vi "Very Large Scan.vi"() -> ()   [LabVIEW 2020]
uses:
  Labview Library/Libraries/ASG8100CY/ASG8100CY.lvlib
  labview_control/LaoJi/NI CTR/NI DAQ Counter.lvlib
  Labview Library/Libraries/Actuator/Libraries/ActuatorXY/ActuatorXY.lvlib
  <vilib>/Utility/file.llb/Write Delimited Spreadsheet (DBL).vi
panel:
  out "Current Position Ref":refnum<vi>
  in  "Tab Control":enum32{"Main", "Page 2", "Debug"}(tab)
  out "Current Position":dbl[](array[numeric])=[99.99927521, 111.2070236, 118.3306351]
  out "Intensity Graph":dbl[][](graph)=[[12413.426204983658, 12199.09700975098, 13100.481023548917, 11916.694144612435, 12119.311516760476, 12635.21319012371, 12600.857673173667, 13200.126884929949, 12592.951932560312, 11969.74510595764, 12757.379319095471, 11664.809418891542, 11252.101294813838, 12673.211709104853, 12762.210663033009, 14052.009205428216, 12767.060980066512, 13491.678523119946, 12391.823407855252, 11682.597991673752, 13135.443159598599, 12561.438316974325, 12594.840161799231, 13137.006262002198, 12816.803806226804, 12264.51133348734, 13282.37239444406, 12068.37184342732, 13200.247759910138, 12739.193364141081, 12895.366092829376, 12574.704114298595, 13495.231009763791, 0.0, 0.0, 0.0, 0.0, 0.0, 0.0, 0.0, 0.0], [13918.401679718641, 13714.354354301113, 13034.107622027206, 12922.275529666118, 13284.51544235071, 13849.07101035678, 14229.907876224646, 12250.565796848681, 14368.52797214958, 11930.191715870234, 11958.175709508474, 13105.942468762929, 13127.623035352512, 13105.907908558916, 12944.940179229601, 12589.116808072462, 11930.893105657193, 12931.543845861952, 12948.5567459181, 13538.329558943446, 12206.628529994818, 12644.786069328475, 12145.374852409574, 13707.10706877193, 14002.386549620609, 13960.120590446573, 14233.993458009523, 12999.121140833002, 12498.726355937248, 13409.675547954475, 13890.523068108716, 13990.040985864322, 0.0, 0.0, 0.0, 0.0, 0.0, 0.0, 0.0, 0.0, 0.0], [12258.885994441494, 11540.699981915297, 12671.034725380556, 13626.04598248154, 12138.002922650432, 13724.579875024094, 13201.121594358172, 13406.793426249373, 12078.138573089063, 12625.023266417908, 11618.085489322053, 12985.45304949292, 13721.167006080777, 13294.601722768217, 12643.786506517528, 12910.677362525515, 12636.198302313776, 13450.034803844776, 13572.657979759677, 12959.536310430212, 14230.075367851714, 13101.468853699516, 13751.366005972177, 14847.158624393935, 14550.879575372923, 13469.328652192455, 12315.062611626825, 13303.949544773273, 12537.014442172915, 13137.644981314217, 12412.402936331515, 12742.456001832838, 0.0, 0.0, 0.0, 0.0, 0.0, 0.0, 0.0, 0.0, 0.0], [12694.372162417198, 13022.362890161545, 12661.942618493797, 13011.002050819809, 12568.862180133716, 12097.617475458834, 11886.783257923727, 13196.39299096777, 12574.726162508628, 13817.079693788166, 12952.933199438578, 11998.72639002685, 12725.850266025853, 12921.012420362225, 13116.183890060925, 12243.709381676368, 13406.677064262141, 12829.310502766873, 12819.63682004765, 14965.923746577075, 14282.102716657535, 14193.667647894785, 14001.343326690692, 14112.343845648364, 14258.49223877884, 13787.255521432566, 13900.845106555598, 13300.272018979244, 14621.216062749454, 13324.138114378447, 12753.532011624226, 13291.486009963373, 0.0, 0.0, 0.0, 0.0, 0.0, 0.0, 0.0, 0.0, 0.0], [12970.08256106479, 12755.433230499591, 12759.129541822067, 12131.866370843865, 13237.441493833365, 13004.551590371122, 12615.955472099551, 12489.827104668824, 13802.62250032107, 13201.604045018365, 13475.38636627498, 13263.586718391252, 12431.667821280345, 12146.212131205706, 11431.705474578237, 11935.857165786505, 13076.264149631565, 14053.653273820904, 13527.554378636914, 15083.728340807605, 14240.050392863022, 13712.466300859343, 13534.211849650283, 13916.161814929561, 13603.915208894614, 12724.175933694143, 14115.521428734177, 13699.377054098575, 12520.16952542519, 13143.571617498012, 12861.319494535608, 11964.754673245552, 0.0, 0.0, 0.0, 0.0, 0.0, 0.0, 0.0, 0.0, 0.0], [12837.099554190312, 13730.039481956715, 13729.236149582926, 12773.22315006938, 12449.36205497966, 12785.572491273708, 12764.465845887613, 12994.325806181272, 12714.702145013536, 13238.071134532476, 12915.19688512138, 13249.255351726322, 14121.254504473844, 12260.006974490901, 12593.537750831047, 13058.366060936138, 12230.519744388814, 13649.845877797894, 14208.99419364147, 13172.418622381581, 14028.88379983732, 14304.007844736365, 12729.821623627164, 14018.217130770625, 12876.63311433904, 13339.02464907911, 13686.55164368562, 12653.270268864537, 11687.751773397524, 14504.962939666611, 13514.353683396563, 12698.999482473548, 0.0, 0.0, 0.0, 0.0, 0.0, 0.0, 0.0, 0.0, 0.0], [13835.660926920731, 11722.788966750355, 13769.097382965234, 13678.968748706233, 13089.742611497875, 13408.31701152738, 12433.082271814066, 13644.416984836844, 12930.603615104978, 13441.534344950353, 12074.964570721304, 13998.007066951823, 13140.736615945742, 11457.928449629886, 13243.337051247401, 13132.571799008621, 13556.25847025227, 13266.56825136083, 13759.25276363223, 13222.940798425003, 12226.586254185257, 12399.172944289516, 12940.666377460031, 12378.023558911598, 12735.176254639584, 13256.409423687672, 12502.46312201368, 12641.192647307607, 13864.041481336862, 10910.96844711718, 12951.07038744892, 13897.890596552874, 0.0, 0.0, 0.0, 0.0, 0.0, 0.0, 0.0, 0.0, 0.0], [13267.677925089234, 14283.60175716499, 12335.566256102135, 13295.740020797984, 13540.983823787685, 13071.811249785284, 13279.048757437493, 12658.988883489092, 14360.12103870256, 12765.068844317735, 12462.974160932763, 13449.15481857287, 12483.51941953124, 13571.643726880155, 12881.600996229157, 11701.869219834029, 13048.415806461859, 12637.200253227616, 13986.802023347125, 12709.817363228733, 13055.41945281852, 12432.331894928056, 12696.068428366405, 12886.427182168558, 12978.607208713736, 12200.297054732728, 13006.564731219401, 12985.287768575094, 13518.967571938578, 12506.537507612435, 11267.832353948912, 11994.032241170093, 0.0, 0.0, 0.0, 0.0, 0.0, 0.0, 0.0, 0.0, 0.0], [13947.00139457789, 13331.572961523247, 12915.551134096198, 12670.150399341737, 13018.4849369988, 13851.488791463342, 12911.337638456574, 12843.950999847997, 13558.792150795012, 12799.452431282652, 12923.843316135377, 13011.771113391505, 12634.113427980472, 14059.777594765874, 12752.741503344181, 13751.440184666115, 11876.017007412478, 12536.136490651717, 12907.728373486574, 11110.785279296422, 12224.148192732144, 12881.137035175328, 11652.240083657447, 12261.757631216198, 12654.62158363913, 12837.346905705253, 13604.085733591222, 12992.350424055434, 12590.268312446482, 13552.180822354245, 13018.53918713744, 13181.501959240637, 0.0, 0.0, 0.0, 0.0, 0.0, 0.0, 0.0, 0.0, 0.0], [12537.114237940512, 12761.908436904923, 12729.829897669371, 13253.403017391156, 13096.430570004553, 14105.53717241387, 11077.027950579277, 12762.431676759352, 13806.015378703643, 12836.928438252402, 12884.267634496216, 12355.610774069048, 12534.66407270051, 13849.386237015919, 14946.701049975214, 12845.299773218543, 11793.55286062109, 13653.118236811586, 12506.03796888722, 12454.347540059242, 11370.323456376876, 12289.249415225073, 11926.627389740292, 12878.692883758606, 13467.001048772585, 13034.782634630774, 13442.312889726498, 13518.001076147912, 14420.255986287922, 12821.079626999623, 12707.021281232992, 12766.684649955621, 0.0, 0.0, 0.0, 0.0, 0.0, 0.0, 0.0, 0.0, 0.0], [12487.381516153826, 14339.319214684385, 12952.083892837984, 13042.298089558928, 11814.040971125112, 12993.245469552056, 11824.266928359524, 12704.546508075906, 12378.064320131107, 13955.37634137259, 13222.720190755503, 12842.786688775011, 12781.837874872224, 14230.39468332686, 13776.254622417897, 12565.57764822756, 12802.501202154437, 13481.234256200964, 13121.367591580052, 12214.942948555188, 12572.122074449308, 12294.665541499931, 11647.169328782516, 13389.589848651389, 13145.55231421336, 13022.516033877246, 12531.205641182538, 12454.90174430176, 13651.922591104285, 13244.0219322327, 13714.922110203477, 13115.428630787026, 0.0, 0.0, 0.0, 0.0, 0.0, 0.0, 0.0, 0.0, 0.0], [13871.946798881001, 13137.465659369618, 12438.056502485917, 12421.185781436325, 12632.60075176157, 12675.161365119719, 12398.995128619465, 13758.94331665558, 12771.263310990475, 12660.486821039187, 12813.183122209603, 12039.442258650037, 13034.033306046578, 13007.094176496232, 12806.719300435076, 13292.78429470634, 11376.872444320257, 13765.106623258476, 12035.178724409687, 13982.013021054343, 13945.65520895236, 12099.577516209834, 12636.400730915822, 12800.802138670857, 13540.83288539829, 12760.59903885621, 12539.225480698393, 14033.338568510966, 12267.604342318273, 12832.589310804566, 12829.312409175322, 12135.672708799944, 0.0, 0.0, 0.0, 0.0, 0.0, 0.0, 0.0, 0.0, 0.0], [12455.858749892846, 12623.133379160781, 12500.86582954595, 12528.366879721654, 11695.349738708808, 13057.094185604197, 12918.713824075225, 13429.752062168367, 13144.681572748195, 14062.331790855842, 14133.900456575315, 13562.371687492217, 13879.543762425294, 13539.298808378722, 12813.118537834911, 11878.981212560637, 12238.440644268509, 13285.492309722144, 12456.477873719256, 11602.41926149364, 14161.420151438455, 13038.032144165492, 12766.45508319012, 12633.416033100453, 11593.70075901844, 12961.846388662292, 11534.410992302064, 12680.87149702491, 12570.498986741186, 12400.744702794887, 12473.300881067033, 11578.738839559071, 0.0, 0.0, 0.0, 0.0, 0.0, 0.0, 0.0, 0.0, 0.0], [13273.618931821715, 13609.664480714086, 12495.912926045647, 11807.334082303123, 13623.978204541841, 12496.801019503186, 13423.36755685845, 13658.982940375161, 13151.711243542646, 13707.132022575093, 15030.21072087198, 14811.975611139635, 13935.041268841054, 13344.116461784426, 13974.194321770477, 13058.07100568908, 11872.978591312276, 12633.960630367956, 13874.030490294443, 13223.140501311796, 13449.693043326033, 12865.093964362582, 14573.210778783121, 12937.89151870477, 13528.587269419117, 12326.29996655928, 13291.441050661637, 12537.612837597128, 12336.303662429049, 13178.792282272538, 12854.311264287297, 11531.867412501098, 0.0, 0.0, 0.0, 0.0, 0.0, 0.0, 0.0, 0.0, 0.0], [13559.475618266475, 12708.238154432383, 13325.441673780018, 12580.807494439696, 12774.39398446758, 13169.667542076919, 12512.951566178062, 13328.069590584042, 14049.434961167764, 14034.014646536674, 14249.950611104257, 13662.509612307922, 13536.090560109578, 13444.830360467091, 12999.22646787052, 14296.542926343876, 13778.174702169568, 13598.705918248295, 12922.431587196003, 12819.663440612918, 14154.671366562798, 11879.250121768884, 12489.774206606979, 13007.187654857686, 12682.65963905539, 13374.869918322547, 13000.101772810256, 11466.189567113694, 11687.54615721876, 13263.679227321192, 12554.14606653799, 12744.765064601508, 0.0, 0.0, 0.0, 0.0, 0.0, 0.0, 0.0, 0.0, 0.0], [12057.281754790905, 13387.018005800162, 12870.58405669512, 11434.570515641148, 13046.61228460777, 12890.555140926346, 14074.4996600198, 13598.584666875637, 13943.588802829441, 14577.02596700239, 14899.311664954468, 14125.407337372551, 13767.921744085745, 14284.758467923384, 15150.342978651532, 13758.234606286367, 15287.521726844541, 14210.937685664203, 13071.850929958635, 13162.13602627519, 13156.529223939751, 13754.827910812202, 14063.703872320904, 12580.05864518567, 12815.970416069284, 13279.850720117265, 14251.8788873906, 15911.396908698733, 12792.9727551923, 14541.243511556966, 12623.955055396002, 12233.341117493372, 0.0, 0.0, 0.0, 0.0, 0.0, 0.0, 0.0, 0.0, 0.0], [12422.400854292599, 13006.101586817997, 12270.677099054536, 12788.713622996089, 13069.934150232626, 13427.738445826217, 13197.712398815935, 14806.48232783516, 14093.664993931981, 15246.832539050914, 13706.140353533836, 15044.001245140858, 14574.332330867643, 15451.759803052615, 14425.683852177626, 14999.999995469241, 14492.149549680014, 14794.979291817484, 14502.670743306082, 13371.240573606086, 13123.269879924728, 13982.645466003423, 11868.955939150304, 13309.303570999804, 12085.546335378644, 13774.74630045686, 12561.019938546375, 14103.989803286822, 12943.419711271907, 14838.47766353947, 12259.99290706767, 13533.39019912427, 0.0, 0.0, 0.0, 0.0, 0.0, 0.0, 0.0, 0.0, 0.0], [12865.076239061886, 12983.967180450174, 13122.511901548021, 13270.715956288306, 13316.070515659632, 14889.493068517446, 14754.714918544232, 15703.222518057488, 15584.692963321164, 15170.03076251474, 15265.426330695644, 14620.072198552392, 14710.705696304709, 14920.583460947415, 15090.151819254193, 15905.83202339489, 14811.806842630936, 14907.515195633481, 13706.047582468886, 14097.047042284901, 13755.202393529396, 14914.267983744412, 13509.689238613517, 13215.87365729284, 14479.769644192691, 13650.401067511768, 14133.66599702661, 14185.046211909372, 13395.981871932736, 13209.642036389812, 13184.931504820266, 11385.65343361341, 0.0, 0.0, 0.0, 0.0, 0.0, 0.0, 0.0, 0.0, 0.0], [12557.855834145807, 12405.97320016197, 13248.758142845036, 12191.34347029364, 14140.106775683014, 14758.926276562219, 15453.21646644145, 15676.658868274886, 14223.4472983029, 16420.85750820729, 14955.950307825911, 15901.80130348282, 15280.378695010344, 15898.304741990773, 15643.332032499364, 16967.81166005398, 15653.588130649729, 14133.05868971342, 13631.134842905734, 15411.594102522207, 14742.377789088294, 14610.103269986652, 13456.5785056317, 13242.281827083545, 14994.206024423704, 14225.606086375425, 14706.421803722222, 15220.649014973435, 12800.431173191871, 13296.491672940598, 13480.498208474472, 12429.374756756852, 0.0, 0.0, 0.0, 0.0, 0.0, 0.0, 0.0, 0.0, 0.0], [12502.114084437491, 12088.404760758222, 13006.384657046532, 13164.00292053339, 13958.505173627442, 14051.552437733617, 13182.061549729364, 15677.026458255068, 15357.841051746631, 14787.809816088495, 16070.697535450803, 16623.275823499192, 14695.645447177383, 16777.92568969485, 14748.60477751724, 15776.157172708974, 15966.767470527393, 14344.047394303958, 15180.2530425606, 14022.757696580164, 14318.918281398463, 14449.611400859467, 13568.738138656865, 14758.521208606704, 13373.508088178725, 13261.572740959322, 14190.787256041518, 13844.008296598327, 13911.94936060347, 12588.100731247758, 14264.334488316377, 12266.928359111278, 0.0, 0.0, 0.0, 0.0, 0.0, 0.0, 0.0, 0.0, 0.0], [12643.366747476926, 11972.530949574875, 13215.254758431174, 14143.841857093452, 12998.965454429928, 13086.238313848029, 15228.324013017324, 15066.738129939753, 16109.733354191218, 15386.56662902939, 16654.96137158211, 17019.565805166, 17304.700496789676, 17078.416436532407, 15632.53884190061, 16197.871133421206, 16829.430171183158, 15584.499221002216, 16292.25163612787, 15966.85228224687, 15275.794506995153, 14030.78736369024, 13084.90193058179, 13254.393049800092, 13753.271002236645, 14077.399983315414, 12308.73432053298, 12926.175679519885, 14349.056090635228, 13604.18653151363, 14535.72137306923, 14496.984491907573, 0.0, 0.0, 0.0, 0.0, 0.0, 0.0, 0.0, 0.0, 0.0], [13370.31128965041, 12977.621033955824, 13245.828564228366, 13493.345323087793, 12392.031485138597, 14437.06914668699, 13851.933787126258, 13990.125805728161, 15128.28720743473, 16031.996202895887, 18481.02026150857, 15242.041644692315, 15475.064201506602, 17548.89108099867, 16827.477646509346, 16001.075702118389, 16024.746412389559, 13721.732727761864, 15622.605805381503, 14467.708881398506, 13811.451629723742, 13880.69199344368, 12927.203687720485, 13349.719588084066, 14861.525356985228, 13272.498346911241, 13202.3354016208, 13737.22916825854, 14822.79564942803, 12780.848688908936, 14063.755691859693, 12791.479310696497, 0.0, 0.0, 0.0, 0.0, 0.0, 0.0, 0.0, 0.0, 0.0], [13517.048924991845, 13100.303643349873, 13839.567226684294, 12142.645485765588, 14453.177249270428, 13688.116915307666, 15547.253147175443, 15954.827490843272, 15715.610837607983, 16690.100248954266, 16737.182882883866, 17332.371926015054, 17483.445469268157, 18032.64214448167, 16258.530707332775, 18352.657472328567, 17106.21525641404, 15463.91752196599, 14996.20028311758, 14695.650700387292, 14185.583457328059, 14440.905008296115, 14744.970853913053, 14118.372997513872, 14936.7181012185, 13771.121924452144, 14314.451070459847, 12855.118432209549, 14354.051659138218, 11967.120500064968, 14193.924072474974, 13247.640785598678, 0.0, 0.0, 0.0, 0.0, 0.0, 0.0, 0.0, 0.0, 0.0], [12293.471357192411, 12226.38799955064, 12455.913516216571, 13132.266009733257, 12515.153790258608, 14031.228647166721, 13407.083294154087, 15968.0, 14507.309454949069, 14583.57069331596, 17753.48118832408, 16535.883876102675, 16794.35978579401, 17636.564434961343, 16603.89990629336, 17441.3154992632, 16269.796786663635, 16473.734108182693, 15696.2257062951, 16975.724388869025, 15210.370341047173, 14811.325017684518, 13664.979709970776, 13856.540583741911, 13489.57623695918, 12631.305501319124, 13405.634386460397, 13359.416003160526, 13953.347283944195, 12697.303672809827, 12462.095868575663, 12778.664271419344, 0.0, 0.0, 0.0, 0.0, 0.0, 0.0, 0.0, 0.0, 0.0], [12739.955228234921, 12252.907673381264, 12801.7679899394, 13294.090413170095, 14134.60390237021, 13991.282354129253, 14271.27311981502, 15407.413222724821, 15513.094778385946, 15822.784812125014, 15958.382134633239, 17960.3805298721, 17428.25201286278, 18646.49192184965, 18010.136260562962, 17987.698732719633, 16621.851214287206, 17419.350675631824, 14746.729957890026, 16777.484940513015, 14663.050448157548, 15149.769193942475, 13594.50468167116, 12971.95571029519, 13366.16250299396, 12349.151681346619, 12725.143669905005, 12272.261648545456, 13121.273709971618, 12879.967441739718, 14028.928847064983, 13068.977678399828, 0.0, 0.0, 0.0, 0.0, 0.0, 0.0, 0.0, 0.0, 0.0], [12492.171790246337, 12551.296234250594, 12523.838945963844, 13092.18518370972, 13189.210632081813, 13993.311673674876, 15138.365318643078, 15881.48765545004, 14969.463622618972, 16971.054736996215, 17380.43377702291, 17703.209709159855, 18240.090037959006, 18556.175213247105, 19058.00821273062, 17323.793468892956, 17680.666059191233, 17778.0737066739, 16422.91368294277, 17404.177001192867, 15637.16410537616, 15125.235586627014, 13553.18135902796, 13446.839145489132, 12768.609994172646, 13309.477355584726, 12447.648129482914, 13631.593915719834, 13284.350702105781, 12139.353126605076, 13480.154400361962, 12872.839321693937, 0.0, 0.0, 0.0, 0.0, 0.0, 0.0, 0.0, 0.0, 0.0], [12501.218197771126, 13324.561608671956, 13544.228395442931, 14816.710555904923, 13244.515887114781, 13765.09746853085, 13594.702454196735, 14350.176707978415, 16495.896145625025, 15799.358089614818, 17181.378087997113, 17537.402994756165, 17962.282492253744, 18119.663872488527, 18263.633347809395, 18213.93801668653, 17843.268935628905, 18433.51645479146, 17704.723103492543, 16231.087584686296, 15342.895878798776, 13927.251761496851, 14212.715865666474, 13157.983069318136, 12595.594549627556, 12725.481646331766, 13662.128444131216, 11230.395636643447, 12706.649815223052, 11858.055682181477, 12769.603673594662, 13256.05472940554, 0.0, 0.0, 0.0, 0.0, 0.0, 0.0, 0.0, 0.0, 0.0], [13857.512544698839, 15709.216972577115, 13848.000592018663, 14110.679397444079, 14756.817814177983, 15096.268528199036, 12735.728593020624, 15320.003168173227, 15090.273969405855, 16005.173919122013, 17046.84089677335, 17393.15289041886, 18125.610479449595, 17787.264316011195, 18970.794026374908, 17624.76965585236, 18281.067410376992, 17661.230722608478, 17205.415389510803, 17345.302984928276, 15212.671105467827, 14688.767236535048, 13946.495567374315, 12844.060685767745, 14040.530987236269, 12518.146398162238, 13168.142994125754, 11890.997005219937, 13168.236986434023, 12623.06657443203, 13513.603693615176, 12036.432468689562, 0.0, 0.0, 0.0, 0.0, 0.0, 0.0, 0.0, 0.0, 0.0], [13097.880192123343, 14864.981970879613, 14627.456956976983, 15552.256928214605, 13415.88917238188, 14236.363461612693, 15100.844916793774, 14324.58574553272, 14207.116537719327, 15266.91659575524, 15376.036476378296, 15405.55198621008, 19277.719226439214, 19088.18477521673, 18259.14035344528, 16354.43568518216, 18061.994943115293, 16189.680383339952, 15352.895826718584, 16828.268842122066, 16167.988698654633, 13773.789233408259, 14189.928754118526, 14367.526706090597, 13246.187950383897, 12517.900594985009, 13030.919715266717, 12732.443078431555, 12235.79495883463, 12999.07149635248, 12005.301542396843, 14455.123105077117, 0.0, 0.0, 0.0, 0.0, 0.0, 0.0, 0.0, 0.0, 0.0], [15246.179965103964, 14126.293675762003, 14031.191647729174, 14275.37329256934, 14816.681877770283, 14557.588893472044, 15688.30788989457, 15037.544288471167, 14222.45101272904, 16366.998724887004, 16421.526389762777, 16420.862637726277, 17119.8488130454, 16819.05262691617, 16177.10235398821, 16385.846391456893, 17035.060610621113, 15480.290211366118, 16175.113479403877, 15480.599207516281, 15536.325493579932, 13836.713632696987, 14908.564031588003, 13717.196582080323, 14121.089185366753, 13685.977604640037, 12703.507919690355, 11598.961746518808, 12696.99762924022, 13991.394101252918, 13340.020054818053, 13616.001980236257, 0.0, 0.0, 0.0, 0.0, 0.0, 0.0, 0.0, 0.0, 0.0], [13348.497950252045, 13506.750167273307, 15028.604443487327, 14246.884724386808, 14043.850657356252, 13900.207677924574, 15267.328915390899, 15791.751767201928, 13885.804993337651, 13930.163446078157, 15603.73273743012, 15300.516986772584, 15471.739280942544, 16342.76219366645, 17728.242759781242, 15403.447926612622, 15525.039055321551, 13232.790721734305, 16693.36707555501, 16196.668202975228, 14115.605511000507, 14334.102073947297, 13834.184535360573, 13883.961471756236, 13733.511707205587, 13118.601385081918, 12431.922343075488, 12413.14001388472, 12252.29604100895, 12440.270750048076, 13576.253284341266, 11599.913926930345, 0.0, 0.0, 0.0, 0.0, 0.0, 0.0, 0.0, 0.0, 0.0], [13729.208643133363, 13505.537267109772, 14952.454555642722, 12824.219742429017, 13948.172205462286, 14768.646225242834, 15143.051353850638, 14688.501299425247, 14210.60110649001, 13442.568131046195, 13605.711100217126, 15635.372330016322, 15971.686857426057, 15354.789714392211, 15062.971126506165, 14566.813116735319, 13300.194803027896, 16243.168211692695, 15535.322671806609, 13612.768577859002, 14605.23411064778, 13027.183819050211, 13723.649400282351, 13395.438482473251, 13091.934101877308, 13302.805954408203, 14096.904415798377, 13461.631139376794, 11324.32201534619, 12200.838651300497, 12664.751235145191, 11712.942296521996, 0.0, 0.0, 0.0, 0.0, 0.0, 0.0, 0.0, 0.0, 0.0], [15029.384806434518, 12569.01736952105, 12846.287523674122, 13173.628422471333, 12887.905670652466, 14366.09601363714, 15233.979154066246, 14600.939878666115, 15520.215253866694, 14334.097817974744, 14761.325334436333, 13450.035484390155, 15354.646500560337, 14764.68778317609, 14904.555301160555, 14029.040110133781, 16387.544164082676, 14799.202471458559, 15024.018662889535, 14995.83075037572, 13420.125581345952, 14816.24848076997, 12784.69624422291, 14188.507311587497, 12794.962400314433, 13284.66673254992, 13554.669363184932, 12495.763419630362, 13922.799084791932, 11726.766342883966, 12733.805008298104, 13625.490774379878, 0.0, 0.0, 0.0, 0.0, 0.0, 0.0, 0.0, 0.0, 0.0], [13727.31503077312, 12282.896552873406, 12993.606742294905, 13184.689656000468, 12685.114166978861, 12564.88216091661, 14120.030322701125, 13648.51032068617, 15312.047857923608, 15928.75268809039, 13705.80473244243, 14340.57159037476, 15814.613995717678, 15144.30647461296, 15688.840229551712, 13648.967072039415, 12962.013565685227, 14799.86318057995, 15426.082509773065, 13895.609640377876, 12950.463641557633, 14589.661495547989, 14854.446588357481, 14610.151893552327, 13295.207049484869, 13549.85940445823, 12465.947921569084, 13438.51208756311, 13113.695743245058, 11811.299477059334, 12788.055827456903, 12920.631843040062, 0.0, 0.0, 0.0, 0.0, 0.0, 0.0, 0.0, 0.0, 0.0], [12804.946825551533, 12791.199653148495, 12071.699812420959, 13917.748703517744, 14236.049170355049, 12523.140583219623, 14135.593218330794, 14016.926350128426, 14782.670899585271, 13977.399254413027, 14945.141189508104, 16076.411828437103, 14750.01444149086, 14732.196699167493, 14139.271832119426, 14085.960995176261, 14305.177111496541, 14257.64952428444, 14344.058172141422, 14803.254030985618, 12904.036974235898, 13383.77647676246, 14250.589598657838, 13180.8856912157, 13834.270131972404, 12623.944177430141, 12899.683461629096, 11931.100401709418, 11859.329608688635, 12815.519762479062, 12735.252931866487, 11843.702928989931, 0.0, 0.0, 0.0, 0.0, 0.0, 0.0, 0.0, 0.0, 0.0], [12957.404586111807, 13666.056251335754, 12980.101503702803, 13188.998346504977, 13127.206869172911, 14144.745660879502, 14050.312859386764, 15716.274822710113, 16041.235603585264, 14735.315637686552, 14984.983065197728, 15420.7910922481, 14813.1073984849, 15540.56799316592, 13642.796874114263, 14362.742429601447, 14840.663418430944, 14491.688977238939, 14224.175705007425, 14071.3259096335, 13661.24837889464, 15026.090761876205, 15260.121626611746, 13753.46334192511, 13705.96708397043, 12838.055241430058, 13377.426777450231, 12404.63106190544, 12733.703890280683, 13024.602027687073, 12480.015108382144, 11631.777053228614, 0.0, 0.0, 0.0, 0.0, 0.0, 0.0, 0.0, 0.0, 0.0], [13002.804843208633, 11811.565261822558, 13489.585009489738, 13811.572545480136, 13302.54419753063, 14220.282092638818, 14689.239132242525, 13064.070167676142, 13965.107572837285, 14460.1323299737, 14568.164861466355, 14574.662758239338, 13479.822798288506, 13532.303298792694, 13056.10095574842, 14442.509120502398, 15247.03913809049, 15083.723142365574, 15233.089918630953, 13259.410173035287, 13127.524042032166, 14663.782789333141, 14458.587662937818, 13538.805881771654, 13571.853268003166, 13217.732697251353, 13544.077857824113, 14047.523485774134, 12554.59064996008, 12026.359142968025, 12307.24916444649, 12116.711290398584, 0.0, 0.0, 0.0, 0.0, 0.0, 0.0, 0.0, 0.0, 0.0], [13222.635289906524, 11091.529371599912, 13004.251650159811, 12852.337155803456, 14024.911234078503, 13591.217981810014, 13793.944896941335, 12951.210306527455, 12949.281982647923, 14055.745620423138, 14044.395893315319, 15416.551159652292, 13513.118446796138, 13280.30066852846, 13652.56574197326, 14650.778114125224, 14976.165381280407, 15812.766128024667, 14269.985464336123, 13641.291932379732, 14942.374695675784, 14058.667517009784, 14206.669659525169, 13652.907534170503, 15058.624562195728, 13640.069067117907, 13035.234632089787, 10818.666763440126, 11304.677389605513, 11759.716226476483, 12100.433601076704, 11103.246776798322, 0.0, 0.0, 0.0, 0.0, 0.0, 0.0, 0.0, 0.0, 0.0], [12645.894926423447, 12482.962444657896, 12076.153979506542, 12662.77656720931, 12794.792006336971, 12355.777956527543, 14132.759393395849, 13598.726756561999, 13736.358552396936, 13877.493136245925, 14506.251967335653, 14208.245512601516, 13972.98556176245, 13635.745381158742, 14767.05691273909, 14805.378724277194, 15834.015833377387, 13517.302141320668, 15438.58245449284, 13395.824913848006, 14824.064394724826, 14845.036338921109, 13350.223134307002, 12718.91204373206, 13342.668799214853, 12785.967484737008, 11633.879760877078, 12180.776869167603, 13092.33853423821, 11411.078997047905, 11698.363197843963, 10903.754834233272, 0.0, 0.0, 0.0, 0.0, 0.0, 0.0, 0.0, 0.0, 0.0], [12762.876532702567, 13762.795366723818, 11916.017978444854, 12386.960953703696, 13156.515184616015, 13124.633795523241, 12944.67675822541, 10643.513263982872, 13206.96084170968, 12076.80714930371, 13954.7771756304, 13330.282621758099, 13880.01277806489, 14093.834373576548, 13585.69592239855, 13462.574042706883, 14746.456093046532, 15411.092592219895, 14793.35426580775, 14648.48649056882, 13936.955379988762, 13237.331327400436, 14454.292055706217, 14312.830772530475, 13258.381066170188, 11968.373655259922, 11928.455200175982, 12776.501995674073, 12735.262754400004, 11778.916736678044, 11382.856259846201, 12790.643025596868, 0.0, 0.0, 0.0, 0.0, 0.0, 0.0, 0.0, 0.0, 0.0], [13135.83545562699, 13463.141813472537, 13303.099015686603, 12086.433056971766, 12390.042434642626, 13095.792063255712, 12981.998291371598, 11827.72134134359, 13314.808382104955, 13008.566207053842, 13867.574526491906, 14878.16079937208, 14060.921713992824, 14044.237671271945, 13406.866004176907, 12793.490351395216, 14926.971628422307, 14568.431249999461, 15010.428470300994, 13720.299050346766, 13390.56362915429, 13164.628559875404, 13031.943261949038, 14671.44895724443, 12978.231819887067, 12770.45031559331, 12044.766378340522, 12134.138631367123, 12158.41820615577, 11684.524463787544, 11831.95958540421, 12009.08249742605, 0.0, 0.0, 0.0, 0.0, 0.0, 0.0, 0.0, 0.0, 0.0]]
  in  "Scan parameter":T1={"Horizontal axis"=0, "Vertical axis"=1, {"horizontal start"=100.0, "horizontal end"=104.0, "horizontal num"=40, "vertical start"=108.0, "vertical end"=112.0, "vertical num"=40}}
  in  "Stop Button":bool
  out "count Rate":dbl=13495.231009763791 format="%#.1f"
  in  "Pause Button":bool
  out "Laser On":bool
  out "Read + Move Time":u32=53
  in  "Sample Rate":dbl=25.0
  in  "Store path":path=path "I:/scan map test"
  out "vertical range":dbl=4.0
  out "horizontal range":dbl=4.0
  out "horizontal step":dbl=0.1
  out "vertical step":dbl=0.1
  out "Horizontal axis":i8(ring) items=["x", "y", "z", ""]
  out "horizontal end":dbl=104.0
  out "vertical end":dbl=112.0
  out "horizontal start":dbl=100.0
  out "vertical start":dbl=108.0
  out "vertical num":u32=40
  out "horizontal num":u32=40
  out "Remain axis":i8(ring)=2 items=["x", "y", "z", ""]
  out "Vertical axis":i8(ring)=1 items=["x", "y", "z", ""]
  in  "Stop Signal Ref":refnum<vi>
  in  "Scanning":refnum<vi>
  in  "Intensity Graph Ref":refnum<vi>
  out "Position After move 2":dbl[](array[numeric]) format="%.6f"
  out "Position After move":dbl[](array[numeric]) format="%.6f"
  out "V goal position":dbl[](array[numeric])=[108.0, 108.1, 108.2, 108.3, 108.4, 108.5, 108.6, 108.7, 108.8, 108.9, 109.0, 109.1, 109.2, 109.3, 109.4, 109.5, 109.6, 109.7, 109.8, 109.9, 110.0, 110.1, 110.2, 110.3, 110.4, 110.5, 110.6, 110.7, 110.8, 110.9, 111.0, 111.1, 111.2, 111.3, 111.4, 111.5, 111.6, 111.7, 111.8, 111.9, 112.0]
  out "H goal position":dbl[](array[numeric])=[100.0, 100.1, 100.2, 100.3, 100.4, 100.5, 100.6, 100.7, 100.8, 100.9, 101.0, 101.1, 101.2, 101.3, 101.4, 101.5, 101.6, 101.7, 101.8, 101.9, 102.0, 102.1, 102.2, 102.3, 102.4, 102.5, 102.6, 102.7, 102.8, 102.9, 103.0, 103.1, 103.2, 103.3, 103.4, 103.5, 103.6, 103.7, 103.8, 103.9, 104.0]
  in  "milliseconds to wait":u32
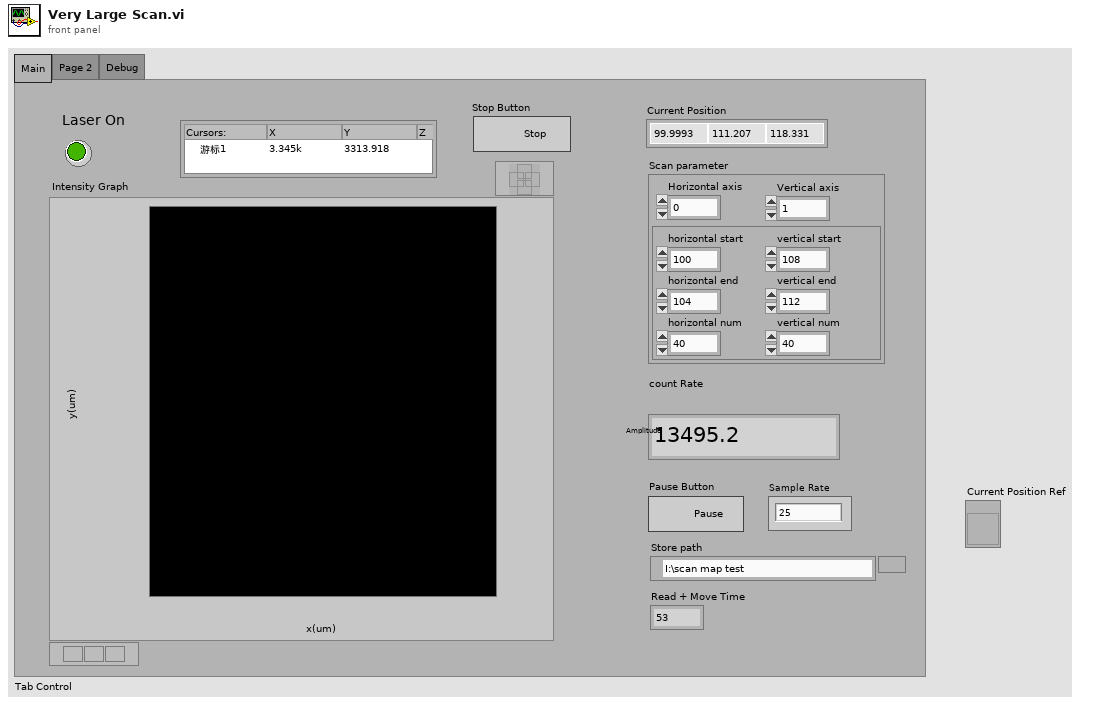
[diagram p1: front panel]
types:
  T1 = cluster{"Horizontal axis":i8, "Vertical axis":i8, cluster{"horizontal start":dbl, "horizontal end":dbl, "horizontal num":u32, "vertical start":dbl, "vertical end":dbl, "vertical num":u32}}
  T2 = enum32{"Bad", "Idle", "Run top level", "Running"}
  T3 = cluster{"horizontal start":dbl, "horizontal end":dbl, "horizontal num":u32, "vertical start":dbl, "vertical end":dbl, "vertical num":u32}
  T4 = typedef "imagedata.ctl" = cluster{"image type":i32, "image depth":i32, "image":u8[], "mask":u8[], "colors":u32[], "Rectangle":cluster{"left":i16, "top":i16, "right":i16, "bottom":i16}}
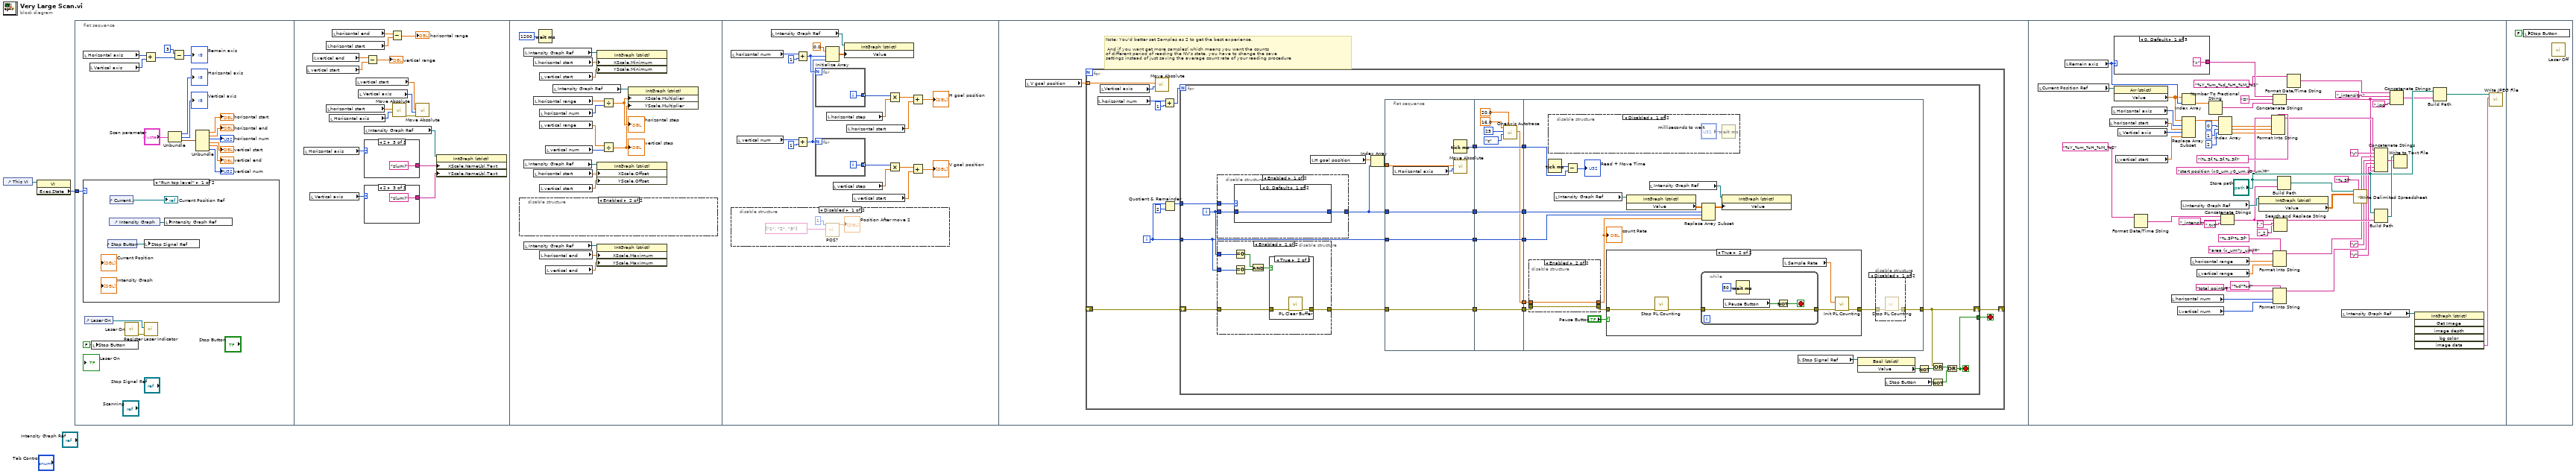
[diagram p0: block diagram]
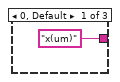
[diagram p3: hidden frame]
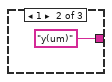
[diagram p4: hidden frame]
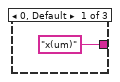
[diagram p5: hidden frame]
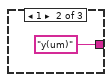
[diagram p6: hidden frame]
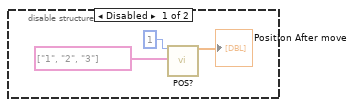
[diagram p7: hidden frame]
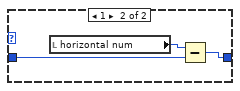
[diagram p9: hidden frame]
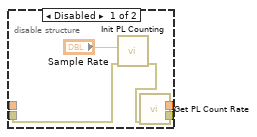
[diagram p14: hidden frame]
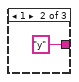
[diagram p17: hidden frame]
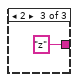
[diagram p18: hidden frame]
diagram:
  n1 = control-ref of="This VI"() -> (w1:refnum<vi>)
  n2 = property class="VI"(reference=w1) -> ("Exec.State"=w2:T2)  [unwired: 1 in, 2 out]
  n3 = flat-sequence {
    tunnel: w2 -> [w6]
    frame #0 {
      n4 = local read "Horizontal axis"() -> (w8:i8)
      n5 = case shown="\"Run top level\"" w6 {
        frame "Run top level" {
          n6 = control-ref of="Stop Button"() -> (w23:refnum<vi>)
          n7 = control-ref of="Intensity Graph"() -> (w24:refnum<vi>)
          n8 = control-ref of="Current Position"() -> (→"Current Position Ref":refnum<vi>)
          n9 = local write "Stop Signal Ref"(w23) -> ()
          n10 = local write "Intensity Graph Ref"(w24) -> ()
        }
        frame "Running", Default {
        }
      }
      n11 = control-ref of="Laser On"() -> (w4:refnum<vi>)
      n12 = local read "Vertical axis"() -> (w9:i8)
      n13 = local write "Stop Button"(FALSE ("Continue?")) -> ()
      n14 = call "Laser On.vi"() -> ("error out"=w3:errorcluster)  [unwired: 11 in]
      n15 = Add(x=w8, y=w9) -> (x+y=w10:i8)
      n16 = call "Register Laser Indicator.vi"("error in"=w3, "Laser Indicator Ref"=w4) -> ()  [unwired: 9 in, 1 out]
      n17 = Unbundle("Scan parameter") -> ("Horizontal axis"=→"Horizontal axis":i8, "Vertical axis"=→"Vertical axis":i8, w15:T3)
      n18 = Subtract(x=3, y=w10) -> (x-y=→"Remain axis":i32)
      n19 = Unbundle(w15) -> ("horizontal start"=→"horizontal start":dbl, "horizontal end"=→"horizontal end":dbl, "horizontal num"=→"horizontal num":u32, "vertical start"=→"vertical start":dbl, "vertical end"=→"vertical end":dbl, "vertical num"=→"vertical num":u32)
    }
    frame #1 {
      n20 = local read "Horizontal axis"() -> (w33:i8)
      n21 = local read "vertical start"() -> (w38:dbl)
      n22 = local read "Vertical axis"() -> (w31:i8)
      n23 = local read "vertical end"() -> (w36:dbl)
      n24 = local read "horizontal start"() -> (w35:dbl)
      n25 = local read "horizontal start"() -> (w27:dbl)
      n26 = local read "Horizontal axis"() -> (w26:i8)
      n27 = local read "horizontal end"() -> (w37:dbl)
      n28 = local read "vertical start"() -> (w28:dbl)
      n29 = local read "Vertical axis"() -> (w29:i8)
      n30 = local read "Intensity Graph Ref"() -> (w34:refnum<vi>)
      n31 = case shown="2" w33 {
        tunnel: ["x(um)" "y(um)" "z(um)"] -> w32
        frame 0, Default {
        }
        frame 1 {
        }
        frame 2 {
        }
      }
      n32 = case shown="2" w31 {
        tunnel: ["x(um)" "y(um)" "z(um)"] -> w30
        frame 0, Default {
        }
        frame 1 {
        }
        frame 2 {
        }
      }
      n33 = Subtract(x=w36, y=w38) -> (x-y=→"vertical range":dbl)
      n34 = Subtract(x=w37, y=w35) -> (x-y=→"horizontal range":dbl)
      n35 = call "Move Absolute.vi"("Axis"=w26, "Goal Position(um)"=w27) -> ("error out"=w25:errorcluster)  [unwired: 8 in, 1 out]
      n36 = call "Move Absolute.vi"("error in"=w25, "Axis"=w29, "Goal Position(um)"=w28) -> ()  [unwired: 7 in, 2 out]
      n37 = property class="IntGraph (strict)"(reference=w34, "XScale.NameLbl.Text"=w32, "YScale.NameLbl.Text"=w30) -> ()  [unwired: 1 in, 2 out]
    }
    frame #2 {
      n38 = disable-structure shown="Enabled" {
        frame Disabled {
          n39 = call "POS?.vi"("System no."=1, "Axes to query"=string[] ["1", "2", "3"] ("String")) -> ("Position"=→"Position After move":dbl[])  [unwired: 3 in, 14 out]
        }
        frame Enabled {
        }
      }
      n40 = local read "Intensity Graph Ref"() -> (w48:refnum<vi>)
      n41 = local read "Intensity Graph Ref"() -> (w58:refnum<vi>)
      n42 = local read "Intensity Graph Ref"() -> (w51:refnum<vi>)
      n43 = local read "horizontal start"() -> (w49:dbl)
      n44 = local read "horizontal range"() -> (w63:dbl)
      n45 = local read "horizontal start"() -> (w55:dbl)
      n46 = Wait (ms)(milliseconds to wait=u32 1200) -> ()  [unwired: 1 out]
      n47 = local read "vertical start"() -> (w47:dbl)
      n48 = local read "horizontal num"() -> (w60:u32)
      n49 = local read "vertical range"() -> (w62:dbl)
      n50 = local read "vertical start"() -> (w54:dbl)
      n51 = local read "horizontal end"() -> (w50:dbl)
      n52 = local read "vertical num"() -> (w61:u32)
      n53 = local read "vertical end"() -> (w52:dbl)
      n54 = local read "Intensity Graph Ref"() -> (w59:refnum<vi>)
      n55 = property class="IntGraph (strict)"(reference=w48, "XScale.Minimum"=w49, "YScale.Minimum"=w47) -> ()  [unwired: 1 in, 2 out]
      n56 = property class="IntGraph (strict)"(reference=w58, "XScale.Offset"=w55, "YScale.Offset"=w54) -> ()  [unwired: 1 in, 2 out]
      n57 = property class="IntGraph (strict)"(reference=w51, "XScale.Maximum"=w50, "YScale.Maximum"=w52) -> ()  [unwired: 1 in, 2 out]
      n58 = Divide(x=w63, y=w60) -> (x/y=w57:dbl)
      "horizontal step" <- w57
      n59 = Divide(x=w62, y=w61) -> (x/y=w56:dbl)
      "vertical step" <- w56
      n60 = property class="IntGraph (strict)"(reference=w59, "XScale.Multiplier"=w57, "YScale.Multiplier"=w56) -> ()  [unwired: 1 in, 2 out]
    }
    frame #3 {
      n61 = local read "horizontal num"() -> (w67:u32)
      n62 = disable-structure shown="Disabled" {
        frame Disabled {
          n63 = call "POS?.vi"("System no."=1, "Axes to query"=string[] ["1", "2", "3"] ("String")) -> ("Position"=→"Position After move 2":dbl[])  [unwired: 3 in, 14 out]
        }
        frame Enabled {
        }
      }
      n64 = local read "vertical num"() -> (w74:u32)
      n65 = local read "Intensity Graph Ref"() -> (w69:refnum<vi>)
      n66 = Add(x=w67, y=1) -> (x+y=w71:u32)
      n67 = Add(x=w74, y=1) -> (x+y=w70:u32)
      n68 = for {
        N: w71 -> [_]
        tunnel: [w90] -> w85 mode=indexing
        i -> [w90]
      }
      n69 = for {
        N: w70 -> [_]
        tunnel: [w89] -> w80 mode=indexing
        i -> [w89]
      }
      n70 = Initialize Array(0.0, w71, w70) -> (w68:dbl[][])
      n71 = local read "horizontal step"() -> (w84:dbl)
      n72 = local read "vertical step"() -> (w79:dbl)
      n73 = property class="IntGraph (strict)"(reference=w69, "Value"=w68) -> ()  [unwired: 1 in, 2 out]
      n74 = local read "horizontal start"() -> (w82:dbl)
      n75 = local read "vertical start"() -> (w77:dbl)
      n76 = Multiply(x=w85, y=w84) -> (x*y=w83:dbl[])
      n77 = Multiply(x=w80, y=w79) -> (x*y=w78:dbl[])
      n78 = Add(x=w83, y=w82) -> (x+y=→"H goal position":dbl[])
      n79 = Add(x=w78, y=w77) -> (x+y=→"V goal position":dbl[])
    }
    frame #4 {
      # "Note: You'd better set Samples as 2 to get the best experience,\n\n And if you want get more samples( which means you want the counts \nof different period of reading the NV's state, you have to change the save \nsettings instead of just saving the average count rate of your reading procedure"
      n80 = local read "V goal position"() -> (w91:dbl[])
      n81 = for {
        tunnel: w91 -> [w92] mode=indexing
        shift-right: [w98] -> _
        shift-left: _ -> [w99]
        i -> [w101]
        stop <- w100 stop-if-true
        n82 = local read "horizontal num"() -> (w96:u32)
        n83 = local read "Vertical axis"() -> (w93:i8)
        n84 = call "Move Absolute.vi"("Axis"=w93, "Goal Position(um)"=w92) -> ()  [unwired: 8 in, 2 out]
        n85 = Add(x=w96, y=1) -> (x+y=w94:u32)
        n86 = Quotient & Remainder(x=w101, y=2) -> (x-y*floor(x/y)=w97:i32)  [unwired: 1 out]
        n87 = for {
          N: w94 -> [_]
          tunnel: w97 -> [w127]
          tunnel: w101 -> [w115]
          tunnel: [w122] -> w100
          shift-right: [w119] -> w98
          shift-left: w99 -> [w117]
          i -> [w118]
          stop <- w122 stop-if-true
          n88 = disable-structure shown="Enabled" {
            disable-tunnel: w127 -> [w130 _]
            disable-tunnel: w118 -> [w129 w135]
            disable-tunnel: [w128 w135] -> w113
            frame Enabled {
              n89 = case shown="0, Default" w130 {
                tunnel: w129 -> [w131 w133]
                tunnel: [w131 w132] -> w128
                frame 0, Default {
                }
                frame 1 {
                  n90 = local read "horizontal num"() -> (w134:u32)
                  n91 = Subtract(x=w134, y=w133) -> (x-y=w132:u32)
                }
              }
            }
            frame Disabled {
            }
          }
          n92 = disable-structure shown="Enabled" {
            disable-tunnel: w115 -> [w140 _]
            disable-tunnel: w118 -> [w139 _]
            disable-tunnel: w117 -> [w137 _]
            disable-tunnel: [w136 _] -> w116
            frame Enabled {
              n93 = Equal To 0?(x=w139) -> (x = 0?=w138:bool)
              n94 = Equal To 0?(x=w140) -> (x = 0?=w141:bool)
              n95 = And(x=w138, y=w141) -> (x .and. y?=w142:bool)
              n96 = case shown="True" w142 {
                tunnel: w137 -> [w143 w145]
                tunnel: [w143 w144] -> w136
                frame False {
                }
                frame True {
                  n97 = call "PL Clear Buffer.vi"("error in"=w145) -> ("error out"=w144:errorcluster)  [unwired: 10 in]
                }
              }
            }
            frame Disabled {
            }
          }
          n98 = local read "H goal position"() -> (w114:dbl[])
          n99 = Index Array(array=w114, index=w113) -> (element=w112:dbl)
          n100 = flat-sequence {
            tunnel: [w151] -> w111
            tunnel: w115 -> [w147]
            tunnel: w113 -> [w148]
            tunnel: w116 -> [w146]
            tunnel: w112 -> [w149]
            tunnel: [w148] -> w108
            tunnel: [w147] -> w106
            tunnel: [w146] -> w104
            tunnel: w111 -> [w160]
            tunnel: [w160] -> w110
            tunnel: [w155] -> w109
            tunnel: w108 -> [w155]
            tunnel: [w154] -> w107
            tunnel: w106 -> [w154]
            tunnel: [w153] -> w105
            tunnel: w104 -> [w153]
            tunnel: [w152] -> w103
            tunnel: w110 -> [w175]
            tunnel: [w162] -> w119
            tunnel: w109 -> [w167]
            tunnel: w107 -> [w166]
            tunnel: w105 -> [w164]
            tunnel: w103 -> [w161]
            frame #0 {
              n101 = local read "Horizontal axis"() -> (w150:i8)
              n102 = Tick Count (ms)() -> (millisecond timer value=w151:u32)
              n103 = call "Move Absolute.vi"("Axis"=w150, "Goal Position(um)"=w149) -> ()  [unwired: 8 in, 2 out]
            }
            frame #1 {
              n104 = call "OneAxis Autotrace.vi"("Sample Rate (Hz)"=20.0, "Axis"=enum16{"x", "y", "z"}."z", "No. of Points"=25, "Diameter"=16.0) -> ("Peak Count"=w152:dbl)  [unwired: 4 in, 3 out]
            }
            frame #2 {
              n105 = disable-structure shown="Enabled" {
                disable-tunnel: [w183 w184] -> w171
                disable-tunnel: [w182 w185] -> w165
                disable-tunnel: w164 -> [w179 w185]
                disable-tunnel: w161 -> [_ w184]
                frame Disabled {
                  n106 = call "Init PL Counting.vi"("error in (no error)"=w179, "Sample Rate (Hz)"="Sample Rate") -> ("error out"=w180:errorcluster)  [unwired: 9 in]
                  n107 = call "Get PL Count Rate.vi"("error in (no error)"=w180) -> ("error out"=w182:errorcluster, "Count Rate"=w183:dbl)  [unwired: 8 in, 1 out]
                }
                frame Enabled {
                }
              }
              "count Rate" <- w171
              n108 = disable-structure shown="Disabled" {
                frame Disabled {
                  n109 = Wait (ms)(milliseconds to wait="milliseconds to wait") -> ()  [unwired: 1 out]
                }
                frame Enabled {
                }
              }
              n110 = Tick Count (ms)() -> (millisecond timer value=w174:u32)
              n111 = local read "Intensity Graph Ref"() -> (w168:refnum<vi>)
              n112 = Subtract(x=w174, y=w175) -> (x-y=→"Read + Move Time":u32)
              n113 = case shown="True" "Pause Button" {
                tunnel: w165 -> [w186 w191]
                tunnel: [w186 w188] -> w163
                frame False {
                }
                frame True {
                  n114 = call "Stop PL Counting.vi"("error in (no error)"=w191) -> ("error out"=w190:errorcluster)  [unwired: 10 in]
                  n115 = while {
                    tunnel: w190 -> [w192]
                    tunnel: [w192] -> w189
                    stop <- w193 stop-if-true
                    n116 = local read "Pause Button"() -> (w194:bool)
                    n117 = Wait (ms)(milliseconds to wait=u32 50) -> ()  [unwired: 1 out]
                    n118 = Not(x=w194) -> (.not. x?=w193:bool)
                  }
                  n119 = local read "Sample Rate"() -> (w187:dbl)
                  n120 = call "Init PL Counting.vi"("error in (no error)"=w189, "Sample Rate (Hz)"=w187) -> ("error out"=w188:errorcluster)  [unwired: 9 in]
                }
              }
              n121 = property class="IntGraph (strict)"(reference=w168) -> ("Value"=w169:dbl[][])  [unwired: 1 in, 2 out]
              n122 = local read "Intensity Graph Ref"() -> (w172:refnum<vi>)
              n123 = Replace Array Subset(array=w169, new element=w171, index (row)=w167, index (col)=w166) -> (w170:dbl[][])
              n124 = property class="IntGraph (strict)"(reference=w172, "Value"=w170) -> ()  [unwired: 1 in, 2 out]
              n125 = disable-structure shown="Disabled" {
                disable-tunnel: w163 -> [w178 _]
                disable-tunnel: [w177 _] -> w162
                frame Disabled {
                  n126 = call "Stop PL Counting.vi"("error in (no error)"=w178) -> ("error out"=w177:errorcluster)  [unwired: 10 in]
                }
                frame Enabled {
                }
              }
            }
          }
          n127 = local read "Stop Signal Ref"() -> (w126:refnum<vi>)
          n128 = property class="Bool (strict)"(reference=w126) -> ("Value"=w125:bool)  [unwired: 1 in, 2 out]
          n129 = local read "Stop Button"() -> (w120:bool)
          n130 = Not(x=w125) -> (.not. x?=w124:bool)
          n131 = Or(x=w119, y=w124) -> (x .or. y?=w123:bool)
          n132 = Not(x=w120) -> (.not. x?=w121:bool)
          n133 = Or(x=w123, y=w121) -> (x .or. y?=w122:bool)
        }
      }
    }
    frame #5 {
      n134 = local read "Current Position Ref"() -> (w198:refnum<vi>)
      n135 = local read "Remain axis"() -> (w254:i8)
      n136 = local read "horizontal start"() -> (w220:dbl)
      n137 = local read "Horizontal axis"() -> (w221:i8)
      n138 = case shown="0, Default" w254 {
        tunnel: ["x" "y" "z"] -> w252
        frame 0, Default {
        }
        frame 1 {
        }
        frame 2 {
        }
      }
      n139 = property class="Arr (strict)"(reference=w198) -> ("Value"=w197:dbl[])  [unwired: 1 in, 2 out]
      n140 = local read "vertical start"() -> (w218:dbl)
      n141 = local read "Vertical axis"() -> (w219:i8)
      n142 = Format Date/Time String(time format string (%c)="%Y_%m_%H_%M_%S") -> (date/time string=w248:string)  [unwired: 2 in]
      n143 = local read "horizontal num"() -> (w204:u32)
      n144 = local read "vertical num"() -> (w205:u32)
      n145 = local read "Intensity Graph Ref"() -> (w245:refnum<vi>)
      n146 = Index Array(array=w197, index=w254) -> (element=w253:dbl)
      n147 = Replace Array Subset(array=w197, new element #1=w220, index #1=w221, new element #2=w218, index #2=w219) -> (w217:dbl[])
      n148 = local read "horizontal range"() -> (w209:dbl)
      n149 = local read "vertical range"() -> (w210:dbl)
      n150 = Number To Fractional String(number=w253) -> (F-format string=w250:string)  [unwired: 3 in]
      n151 = Index Array(array=w217, index #1=0 ("index"), index #2=1 ("index"), index #3=2 ("index")) -> (element #1=w222:dbl, element #2=w223:dbl, element #3=w224:dbl)
      n152 = Concatenate Strings(w248, "_intensity" ("string"), ".txt" ("string")) -> (w239:string)
      n153 = property class="IntGraph (strict)"(reference=w245) -> ("Value"=w243:dbl[][])  [unwired: 1 in, 2 out]
      n154 = Format Into String(format string="(%.3f,%.3f,%.3f)", initial string="start position (x0_um,y0_um,z0_um)=" ("string"), w222, w223, w224) -> (resulting string=w213:string)  [unwired: 1 in, 1 out]
      n155 = Concatenate Strings(w252, "=" ("string"), w250) -> (w200:string)
      n156 = Format Into String(format string="%.3f*%.3f", initial string="area (x_um*y_um)=" ("string"), w209, w210) -> (resulting string=w203:string)  [unwired: 1 in, 1 out]
      n157 = Format Into String(format string="%d*%d", initial string="total points=" ("string"), w204, w205) -> (resulting string=w201:string)  [unwired: 1 in, 1 out]
      n158 = Search and Replace String(input string=w239, search string="." ("substring (\"\")"), replace string="_2." ("replace string (\"\")")) -> (result string=w238:string)  [unwired: 1 in, 7 out]
      n159 = Build Path(base path="Store path", name or relative path=w239) -> (appended path=w242:path)
      n160 = Format Date/Time String(time format string (%c)="%Y_%m_%d_%H_%M_%S") -> (date/time string=w234:string)  [unwired: 2 in]
      n161 = local read "Intensity Graph Ref"() -> (w231:refnum<vi>)
      n162 = call-poly <vilib>:"Write Delimited Spreadsheet.vi"("file path (dialog if empty)"=w242, "format (%.3f)"="%.3f", "2D data"=w243) -> ()  [unwired: 11 in, 2 out]
      n163 = Concatenate Strings(w213, "\r", w203, "\r", w201, "\r", w200) -> (w236:string)
      n164 = Build Path(base path="Store path", name or relative path=w238) -> (appended path=w237:path)
      n165 = Concatenate Strings(w234, "_intensity " ("string"), w200, ".jpg" ("string")) -> (w227:string)
      n166 = Write to Text File(file (use dialog)=w237, text=w236) -> ()  [unwired: 1 in, 4 out]
      n167 = invoke class="IntGraph (strict)" method="Get Image"(reference=w231) -> ("image data"=w230:T4)  [unwired: 5 in, 5 out]
      n168 = Build Path(base path="Store path", name or relative path=w227) -> (appended path=w228:path)
      n169 = call <vilib>:"Write JPEG File.vi"("image data"=w230, "path to JPEG file"=w228) -> ()  [unwired: 1 in, 9 out]
    }
    frame #6 {
      n170 = local write "Stop Button"(FALSE ("Continue?")) -> ()
      n171 = call "Laser Off.vi"() -> ()  [unwired: 11 in, 1 out]
    }
  }
